vi "Read (No Check) String.vi"(7 "count":u64 format="%d bytes", 8 "error in (no error)":errorcluster, 9 "offset (0)":u64 format="%d bytes", 10 "buffer in":string, 11 "Pointer in":refnum<class "Pointer.lvclass">) -> (0 "error out":errorcluster, 1 "offset out":u64 format="%d bytes", 2 "buffer out":string, 3 "Pointer out":refnum<class "Pointer.lvclass">)   [LabVIEW 2020, in "Memory Manager.lvlib" / "Pointer.lvclass"]
doc: "Reads <b>count</b> bytes from the address specified by <b>pointer + offset</b> into the provided <b>buffer</b>.\n\n<b>Note:</b> This VI is <b>unsafe</b>.\n\nUnsafe means that it does not evaluate the size parameter of <b>pointer</b> to ensure that is inbounds of allocated memory before peforming a memory read/write. Reading/writing more data to a pointer than it has allocated can corrupt or crash LabVIEW. Only use this VI in scenarios where the <b>pointer</b> has been validated to be allocated to a correct size before calling this VI."
uses:
  Pointer.lvclass
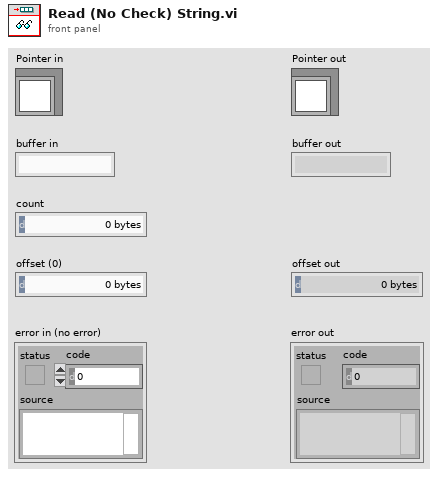
[diagram p1: front panel]
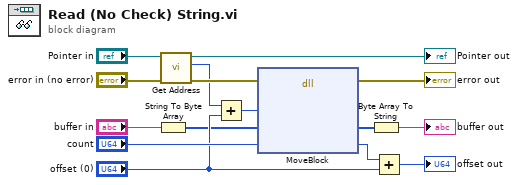
[diagram p0: block diagram]
diagram:
  n1 = String To Byte Array(string="buffer in") -> (unsigned byte array=w2:u8[])
  n2 = call "Get Address.vi"("Pointer in"="Pointer in") -> ("address"=w8:u64, "Pointer out"=→"Pointer out":refnum<class "Pointer.lvclass">)  [unwired: 9 in]
  n3 = Add(x=w8, y="offset (0)") -> (x+y=w10:u64)
  n4 = dll-call lib="LabVIEW" fn="MoveBlock"(error in="error in (no error)", "src"=w10, "dst"=w2, "size"="count") -> (error out=→"error out":errorcluster, "dst"=w11:u8[], "size"=w5:u64)  [unwired: 4 in, 1 out]
  n5 = Byte Array To String(unsigned byte array=w11) -> (string=→"buffer out":string)
  n6 = Add(x=w5, y="offset (0)") -> (x+y=→"offset out":u64)
